vi "Set Temperature and Rise Time2023.vi"(3 "error in":errorcluster, 4 "Slew Time String":string, 5 "Temperature String":string, 6 "Device":cluster{"GPIB #":u8, "Address":u8}={"GPIB #"=0, "Address"=28}) -> (0 "error out":errorcluster)   [LabVIEW 2024]
panel:
  # "Input"
  # "Celsius"
  # "minutes"
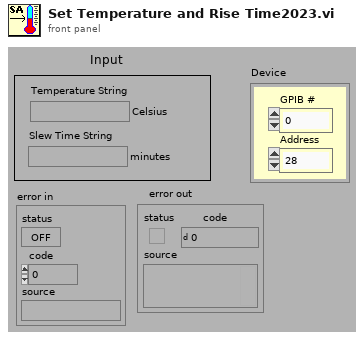
[diagram p1: front panel]
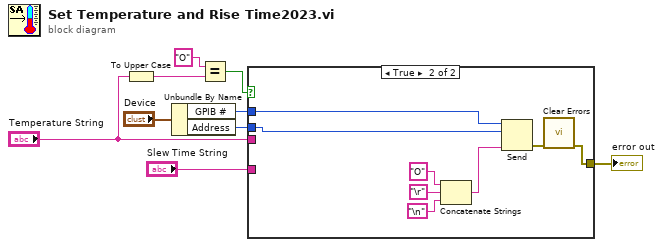
[diagram p0: block diagram]
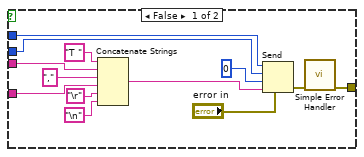
[diagram p2: hidden frame]
diagram:
  n1 = To Upper Case(1:"Temperature String") -> (0:w8:string)
  n2 = Unbundle By Name("Device") -> ("GPIB #"=w3:u8, "Address"=w2:u8)
  n3 = Equal?(x="O", y=w8) -> (x = y?=w6:bool)
  n4 = case shown="True" w6 {
    tunnel: "Temperature String" -> [w16 _]
    tunnel: w2 -> [w15 w25]
    tunnel: [w14 w23] -> w5
    tunnel: w3 -> [w13 w26]
    tunnel: "Slew Time String" -> [w10 _]
    frame False {
      n5 = Concatenate Strings("T " ("Substring"), w16, ",", w10, "\r", "\n") -> (w20:string)
      n6 = Send(0:w13, 2:w15, 3:i16 0 ("mode"), 4:"error in", 5:w20) -> (8:w17:errorcluster)  [unwired: 2 out]
      n7 = call <vilib>:"Simple Error Handler.vi"("error in (no error)"=w17) -> ("error out"=w14:errorcluster)  [unwired: 4 in, 4 out]
    }
    frame True {
      n8 = Concatenate Strings("O" ("data string"), "\r", "\n") -> (w29:string)
      n9 = Send(0:w26, 2:w25, 5:w29) -> (8:w24:errorcluster)  [unwired: 2 in, 2 out]
      n10 = call <vilib>:"Clear Errors.vi"("error in (no error)"=w24) -> ("error out"=w23:errorcluster)  [unwired: 5 in, 1 out]
    }
  }
  "error out" <- w5
